vi "port_iinit.vi"(8 "Timeout (ms)":u32=1000, 11 "VISA Refnum in":refnum<visa-resource-name>) -> (0 "error out":errorcluster, 3 "VISA Refnum out":refnum<visa-resource-name>)   [LabVIEW 2024]
uses:
  <vilib>/Instr/_visa.llb/VISA Configure Serial Port (Instr).vi
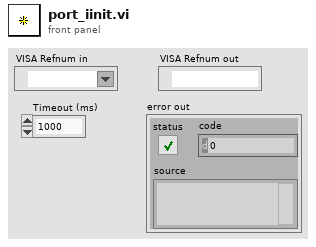
[diagram p1: front panel]
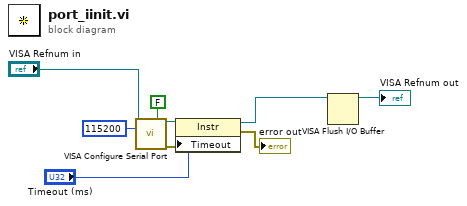
[diagram p0: block diagram]
diagram:
  n1 = call-poly "VISA Configure Serial Port"("VISA resource name"="VISA Refnum in", "Enable Termination\nChar (T)"=FALSE ("Enable Termination\nChar (T)"), "baud rate (9600)"=u32 115200) -> ("VISA resource name out"=w6:refnum<visa-resource-name>, "error out"=w7:errorcluster)  [unwired: 11 in]
  n2 = property class="Instr"(reference=w6, error in=w7, "Timeout"="Timeout (ms)") -> (reference out=w2:refnum<visa-resource-name>, error out=→"error out":errorcluster)
  n3 = VISA Flush I/O Buffer(VISA resource name=w2) -> (VISA resource name out=→"VISA Refnum out":refnum<visa-resource-name>)  [unwired: 2 in, 1 out]
